vi "add.vi"(8 "error in (no error)":errorcluster, 10 "Memento.lvclass":refnum<class "Memento.lvclass">, 11 "CareTaker in":refnum<class "CareTaker.lvclass">) -> (0 "error out":errorcluster, 3 "CareTaker out":refnum<class "CareTaker.lvclass">)   [LabVIEW 2018, in "CareTaker.lvclass"]
uses:
  CareTaker.lvclass
  Memento Class/Memento.lvclass
  CareTaker.lvclass/CareTaker.ctl
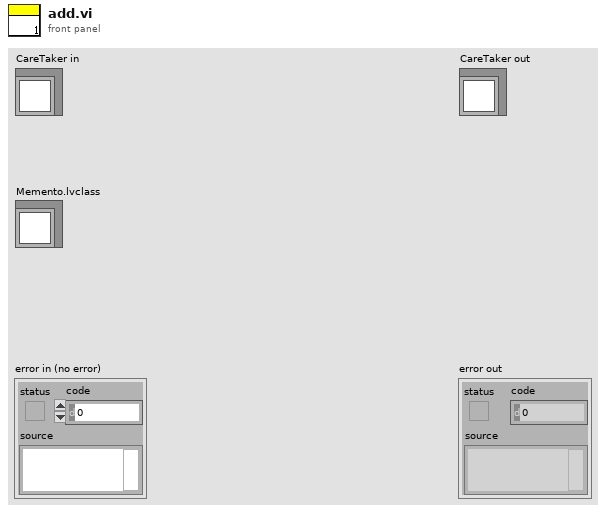
[diagram p1: front panel]
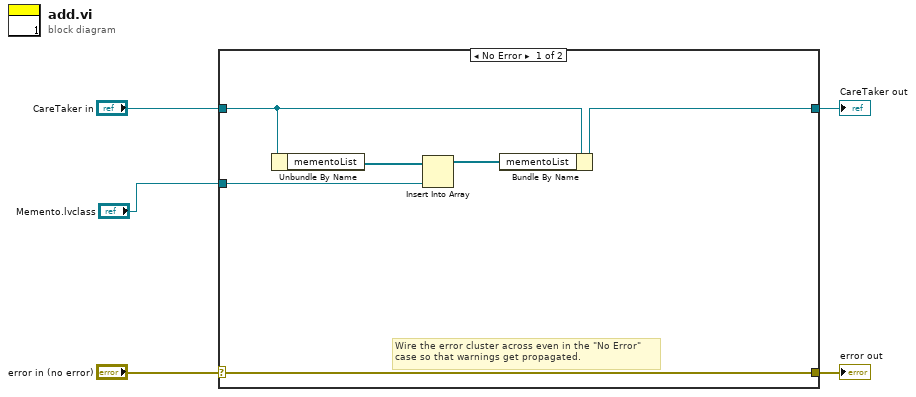
[diagram p0: block diagram]
diagram:
  n1 = case shown="No Error" "error in (no error)" {
    selector: "error in (no error)" -> [w11 w13]
    tunnel: [w11 w13] -> w4
    tunnel: [w9 w12] -> w2
    tunnel: "CareTaker in" -> [w10 w12]
    tunnel: "Memento.lvclass" -> [w6 _]
    frame No Error {
      # "Wire the error cluster across even in the \"No Error\"\ncase so that warnings get propagated."
      n2 = Unbundle By Name(w10) -> ("mementoList"=w8:refnum<class "Memento.lvclass">[])
      n3 = Insert Into Array(array=w8, new element=w6) -> (w7:refnum<class "Memento.lvclass">[])  [unwired: 1 in]
      n4 = Bundle By Name(cluster=w10, "mementoList"=w7) -> (w9:refnum<class "CareTaker.lvclass">)
    }
    frame Error {
    }
  }
  "error out" <- w4
  "CareTaker out" <- w2
